vi "JTAG Read DCO Trim.vi"(8 "error in (no error)":errorcluster) -> (0 "error out":errorcluster, 2 "Trim String":string="Trim Values:")   [LabVIEW 2010]
panel:
  out "Block Contents":u8[](array[numeric]) format="%.0x"
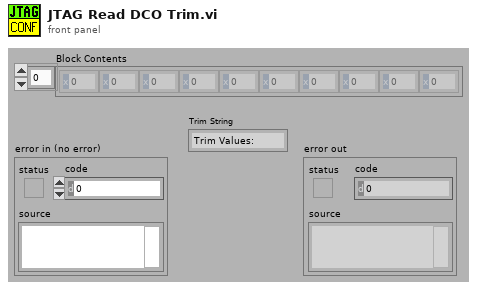
[diagram p1: front panel]
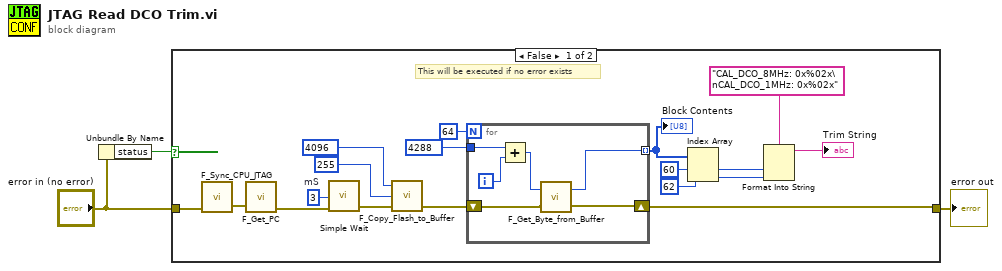
[diagram p0: block diagram]
diagram:
  n1 = Unbundle By Name("error in (no error)") -> ("status"=w2:bool)
  n2 = case shown="False" w2 {
    tunnel: [w13 w28] -> w3
    tunnel: "error in (no error)" -> [w17 w28]
    frame False {
      w21 = u32 3  # mS
      # "This will be executed if no error exists"
      n3 = call "F_Sync_CPU_JTAG.vi"("error in (no error)"=w17) -> ("error out"=w16:errorcluster)  [unwired: 1 in, 1 out]
      n4 = call "F_Get_PC.vi"("error in (no error)"=w16) -> ("error out"=w15:errorcluster)  [unwired: 1 in, 1 out]
      n5 = call "Simple Wait.vi"("mS"=w21, "error in"=w15) -> ("error out"=w20:errorcluster)  [unwired: 12 in, 1 out]
      n6 = call "F_Copy_Flash_to_Buffer.vi"("error in (no error)"=w20, "Block size to be copied"=255, "Buffer start address"=4096) -> ("error out"=w18:errorcluster)  [unwired: 2 in]
      n7 = for {
        N: 64 -> [_]
        tunnel: 4288 -> [w24]
        shift-right: [w26] -> w13
        shift-left: w18 -> [w27]
        tunnel: [w22] -> w12 mode=indexing
        i -> [w23]
        n8 = Add(x=w24, y=w23) -> (x+y=w25:i32)
        n9 = call "F_Get_Byte_from_Buffer.vi"("error in (no error)"=w27, "Address of byte to be read"=w25) -> ("error out"=w26:errorcluster, "Current value"=w22:u8)
      }
      "Block Contents" <- w12
      n10 = Index Array(array=w12, index #1=60 ("index"), index #2=62 ("index")) -> (element #1=w8:u8, element #2=w7:u8)
      n11 = Format Into String(format string="CAL_DCO_8MHz: 0x%02x\nCAL_DCO_1MHz: 0x%02x", w8, w7) -> (resulting string=→"Trim String":string)  [unwired: 2 in, 1 out]
    }
    frame True {
      # "Error exists, skip all functions"
    }
  }
  "error out" <- w3
